vi "4Pi 4Pi Modes - Confirm New Frame.vi"(0 "Camera Notifier Name":string, 11 "Error In":errorcluster, 13 "Wait No. (1)":u32=1) -> (4 "Camera Notifier Name (Dup)":string, 15 "Error Out":errorcluster)   [LabVIEW 2016]
uses:
  Device Library/Cameras/Camera Controls/Generic Camera Actions.ctl
  Device Library/Cameras/Camera Controls/Camera IMAQ Key Info.ctl
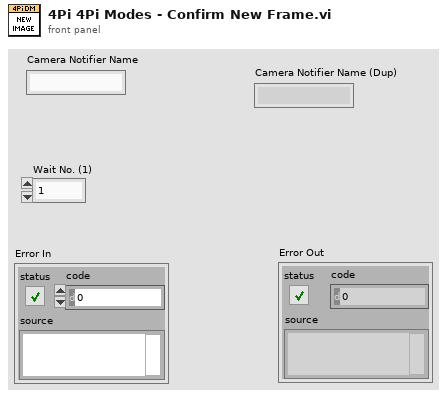
[diagram p1: front panel]
types:
  T1 = typedef "Generic Camera Actions.ctl" = enum16{"Status", "Live Preview", "Capture", "Abort", "Set Exposure Time (s)", "Get Exposure Time (s)", "Record Settings", "Set ROI", "Get ROI", "Defect Correction On/Off", "Cooler On/Off", "Fan On/Off", "Quti"}
  T2 = typedef "Camera IMAQ Key Info.ctl" = cluster{"Frame":u32, "Sensor Height":i32, "Sensor Width":i32, "ROI Height":i32, "ROI Width":i32, "ROI Enable?":bool, "Bit per Pixel":u8}
  T3 = typedef "IMAQ Image.ctl" = refnum<image>
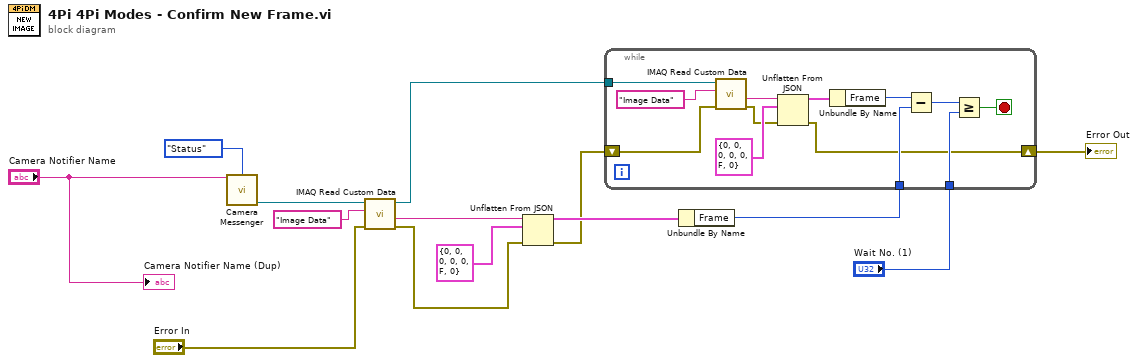
[diagram p0: block diagram]
diagram:
  n1 = call "Camera Messenger.vi"("Notifier Name"="Camera Notifier Name", "General Camera Actions"=Generic_Camera_Actions."Status") -> ("Image Ref"=w10:T3)  [unwired: 8 in, 5 out]
  n2 = call "IMAQ Read Custom Data"("error in (no error)"="Error In", "Key"="Image Data", "Image"=w10) -> ("error out"=w4:errorcluster, "Custom Data Out"=w12:string, "Image (duplicate)"=w9:T3)  [unwired: 6 in]
  n3 = Unflatten From JSON(JSON string=w12, type and defaults=T2 {"Frame"=0, "Sensor Height"=0, "Sensor Width"=0, "ROI Height"=0, "ROI Width"=0, "ROI Enable?"=FALSE, "Bit per Pixel"=0} ("Camera IMAQ Key Info"), error in (no error)=w4) -> (value=w14:T2, error out=w3:errorcluster)  [unwired: 4 in]
  n4 = Unbundle By Name(w14) -> ("Frame"=w8:u32)
  n5 = while {
    tunnel: w9 -> [w23]
    tunnel: w8 -> [w21]
    tunnel: "Wait No. (1)" -> [w18]
    shift-right: [w15] -> w2
    shift-left: w3 -> [w17]
    stop <- w19 stop-if-true
    n6 = call "IMAQ Read Custom Data"("error in (no error)"=w17, "Key"="Image Data", "Image"=w23) -> ("error out"=w16:errorcluster, "Custom Data Out"=w25:string)  [unwired: 6 in, 1 out]
    n7 = Unflatten From JSON(JSON string=w25, type and defaults=T2 {"Frame"=0, "Sensor Height"=0, "Sensor Width"=0, "ROI Height"=0, "ROI Width"=0, "ROI Enable?"=FALSE, "Bit per Pixel"=0} ("Camera IMAQ Key Info"), error in (no error)=w16) -> (value=w27:T2, error out=w15:errorcluster)  [unwired: 4 in]
    n8 = Unbundle By Name(w27) -> ("Frame"=w22:u32)
    n9 = Subtract(x=w22, y=w21) -> (x-y=w20:u32)
    n10 = Greater Or Equal?(x=w20, y=w18) -> (x >= y?=w19:bool)
  }
  "Error Out" <- w2
  "Camera Notifier Name (Dup)" <- "Camera Notifier Name"
